vi "flattenMassToXML_Scalar.vi"(8 "error in (no error)":errorcluster, 9 "massUnitInXML":T1, 10 "massAgain":variant, 11 "mass":dbl[unit]) -> (0 "error out":errorcluster, 3 "xmlString":string)   [LabVIEW 2012, in "UnitsAndXML.lvlib"]
uses:
  <userlib>/Common/UnitsAndXML/UnitsAndXML.lvlib
  <userlib>/Common/UnitsAndXML/FlattenItemWithUnitToXML/FlattenMassToXML/MassUnit.ctl
  <vilib>/Utility/VariantDataType/VariantType.lvlib
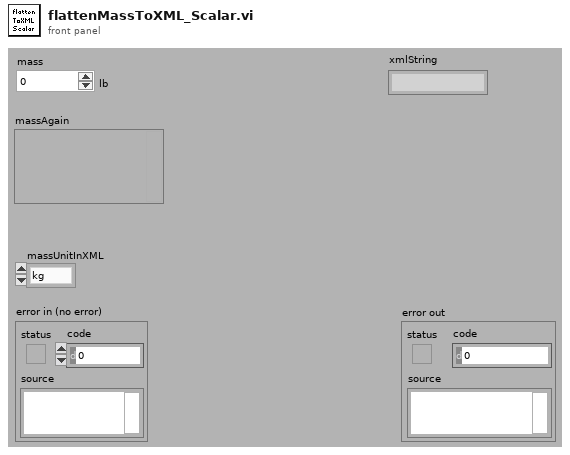
[diagram p1: front panel]
types:
  T1 = typedef "UnitsAndXML.lvlib/MassUnit.ctl" = enum16{"kg", "CM", "dr", "gr", "t", "oz", "lb", "slug", "stone", "Ton", "ton", "u"}
  T2 = typedef "VariantType.lvlib/Type.ctl" = enum8{"Invalid Type", "Void", "I8", "I16", "I32", "I64", "U8", "U16", "U32", "U64", "Single Float", "Double Float", "Extended Float", "Single Complex", "Double Complex", "Extended Complex", "Enum U8", "Enum U16", "Enum U32", "Enum U64", "Single Float With Unit", "Double Float With Unit", "Extended Float With Unit", "Single Complex with Unit", "Double Complex with Unit", "Extended Complex with Unit", "Boolean", "String", "Path", "Picture", "Tag", "Array", "Cluster", "Variant", "LV Variant", "Waveform", "Timestamp", "Digital Waveform", "Digital Data", "ExpressData", "Refnum", "External Data", "VI", "Poly VI", "LabVIEW Class Instance", "Fixed Point"}
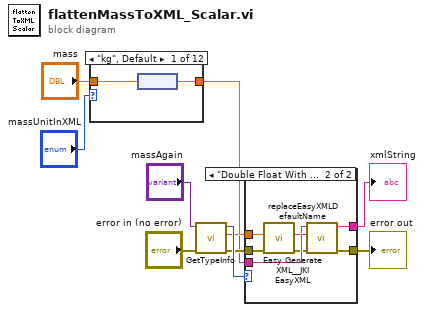
[diagram p0: block diagram]
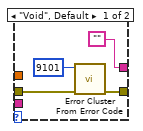
[diagram p2: hidden frame]
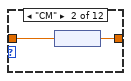
[diagram p3: hidden frame]
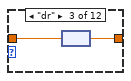
[diagram p4: hidden frame]
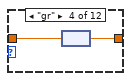
[diagram p5: hidden frame]
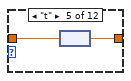
[diagram p6: hidden frame]
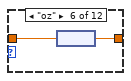
[diagram p7: hidden frame]
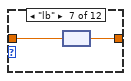
[diagram p8: hidden frame]
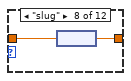
[diagram p9: hidden frame]
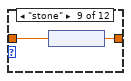
[diagram p10: hidden frame]
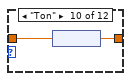
[diagram p11: hidden frame]
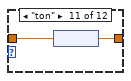
[diagram p12: hidden frame]
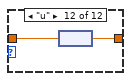
[diagram p13: hidden frame]
diagram:
  n1 = case shown="\"kg\", Default" "massUnitInXML" {
    tunnel: "mass" -> [w12 w14 w16 w18 w20 w22 w24 w26 w28 w30 w32 w34]
    tunnel: [w11 w13 w15 w17 w19 w21 w23 w25 w27 w29 w31 w33] -> w10
    frame "kg", Default {
      n2 = node(w12) -> (w11:dbl)
    }
    frame "CM" {
      n3 = node(w14) -> (w13:dbl)
    }
    frame "dr" {
      n4 = node(w16) -> (w15:dbl)
    }
    frame "gr" {
      n5 = node(w18) -> (w17:dbl)
    }
    frame "t" {
      n6 = node(w20) -> (w19:dbl)
    }
    frame "oz" {
      n7 = node(w22) -> (w21:dbl)
    }
    frame "lb" {
      n8 = node(w24) -> (w23:dbl)
    }
    frame "slug" {
      n9 = node(w26) -> (w25:dbl)
    }
    frame "stone" {
      n10 = node(w28) -> (w27:dbl)
    }
    frame "Ton" {
      n11 = node(w30) -> (w29:dbl)
    }
    frame "ton" {
      n12 = node(w32) -> (w31:dbl)
    }
    frame "u" {
      n13 = node(w34) -> (w33:dbl)
    }
  }
  n14 = call <vilib>:"GetTypeInfo.vi"("error in (no error)"="error in (no error)", "Variant"="massAgain") -> ("error out"=w2:errorcluster, "Name"=w1:string, "Type Enum"=w3:T2)  [unwired: 5 in, 2 out]
  n15 = case shown="\"Double Float With Unit\"" w3 {
    tunnel: w10 -> [_ w45]
    tunnel: ["" w44] -> w7
    tunnel: [w37 w43] -> w6
    tunnel: w2 -> [w35 w40]
    tunnel: w1 -> [_ w42]
    frame "Void", Default {
      n16 = call <vilib>:"Error Cluster From Error Code.vi"("error in (no error)"=w35, "error code (0)"=9101) -> ("error out"=w37:errorcluster)  [unwired: 7 in]
    }
    frame "Double Float With Unit" {
      n17 = call <vilib>:"Easy Generate XML__JKI EasyXML.vi"("error in (no error)"=w40, "LabVIEW Data"=w45) -> ("error out"=w39:errorcluster, "XML String"=w41:string)  [unwired: 8 in]
      n18 = call <userlib>:"replaceEasyXMLDefaultName.vi"("error in"=w39, "desiredName"=w42, "easyXMLStringWithDefaultNames"=w41) -> ("error out"=w43:errorcluster, "xmlString"=w44:string)  [unwired: 7 in]
    }
  }
  "xmlString" <- w7
  "error out" <- w6
